vi "Otm Ref_1.vi"() -> ()   [LabVIEW 2017]
uses:
  Channel Config Cluster.ctl
  Channel Cluster.ctl
panel:
  in  "Array":T1[](array[typedef])
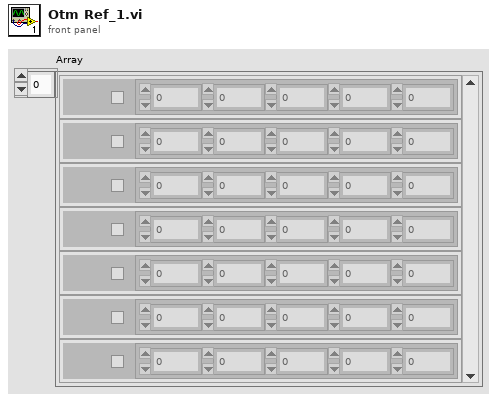
[diagram p1: front panel]
types:
  T1 = typedef "Channel Config Cluster.ctl" = cluster{"chEn":bool, "ptArray":T2, "chName":string}
  T2 = typedef "Channel Cluster.ctl" = dbl[]
  T3 = enum8{"Enabled", "Disabled", "Disabled and Grayed Out"}
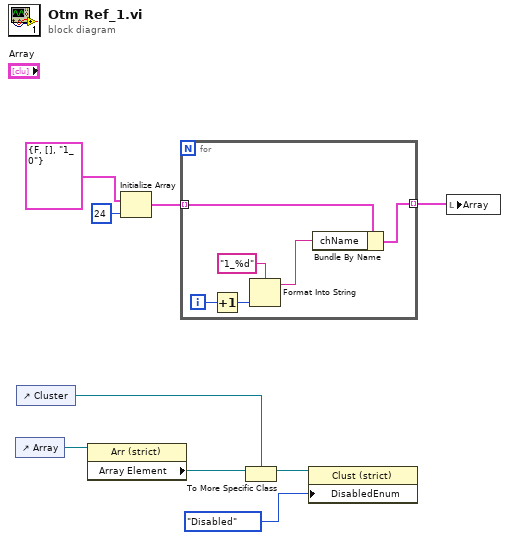
[diagram p0: block diagram]
diagram:
  n1 = control-ref of="Array"() -> (w5:refnum<vi>)
  n2 = control-ref of="Cluster"() -> (w3:refnum<vi>)
  n3 = property class="Arr (strict)"(reference=w5) -> ("Array Element"=w4:refnum<vi>)  [unwired: 1 in, 2 out]
  n4 = Initialize Array(T1 {"chEn"=FALSE, "ptArray"=[], "chName"="1_0"} ("Cluster"), 24 ("dimension size")) -> (w7:T1[])
  n5 = for {
    tunnel: w7 -> [w11] mode=indexing
    tunnel: [w12] -> w6 mode=indexing
    i -> [w14]
    n6 = Increment(x=w14) -> (x+1=w10:i32)
    n7 = Format Into String(format string="1_%d", w10) -> (resulting string=w13:string)  [unwired: 2 in, 1 out]
    n8 = Bundle By Name(cluster=w11, "chName"=w13) -> (w12:T1)
  }
  n9 = To More Specific Class(target class=w3, reference=w4) -> (specific class reference=w2:refnum<vi>)  [unwired: 1 in, 1 out]
  n10 = property class="Clust (strict)"(reference=w2, "DisabledEnum"=T3."Disabled" ("Disabled")) -> ()  [unwired: 1 in, 2 out]
  n11 = local write "Array"(w6) -> ()
